vi "Init.vi"(7 "Enabled":bool, 8 "error in (no error)":errorcluster, 10 "Item ID":i32, 11 "Scene Name":string) -> (0 "error out":errorcluster, 3 "SetSceneItemEnabled out":refnum<class "SetSceneItemEnabled.lvclass">)   [LabVIEW 2020, in "obs-websocket.lvlib" / "SetSceneItemEnabled.lvclass"]
uses:
  SetSceneItemEnabled.lvclass
  SetSceneItemEnabled.lvclass/SetSceneItemEnabled.ctl
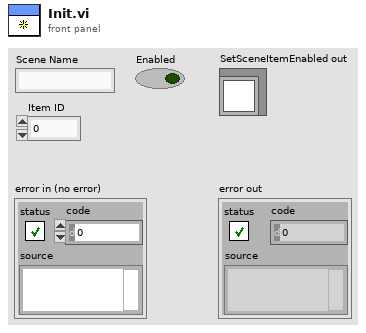
[diagram p1: front panel]
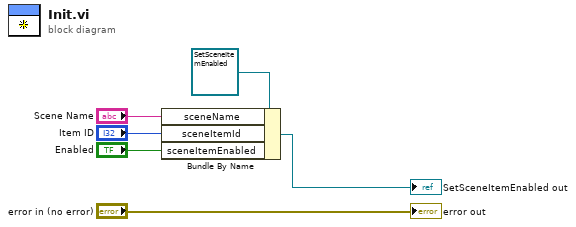
[diagram p0: block diagram]
diagram:
  n1 = Bundle By Name(cluster=refnum<class "SetSceneItemEnabled.lvclass"> refnum ("SetSceneItemEnabled in"), "sceneName"="Scene Name", "sceneItemId"="Item ID", "sceneItemEnabled"="Enabled") -> (→"SetSceneItemEnabled out":refnum<class "SetSceneItemEnabled.lvclass">)
  "error out" <- "error in (no error)"
